vi "rstring.vi"(1 "number":i16) -> (0 "concatenated string":string)   [LabVIEW 2017]
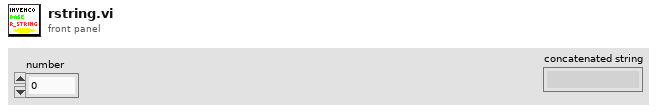
[diagram p1: front panel]
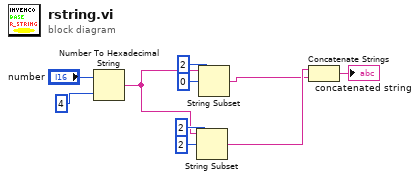
[diagram p0: block diagram]
diagram:
  n1 = Number To Hexadecimal String(1:i16 4 ("width (-)"), 2:"number") -> (0:w3:string)
  n2 = String Subset(string=w3, offset (0)=2, length (rest)=2 ("length (rest)")) -> (substring=w5:string)
  n3 = String Subset(string=w3, offset (0)=0, length (rest)=2 ("length (rest)")) -> (substring=w4:string)
  n4 = Concatenate Strings(w5, w4) -> (→"concatenated string":string)
